vi "Create All Message Queues.vi"(8 "error in (no error)":errorcluster, 10 "Master Queue In":refnum<queue>) -> (0 "error out":errorcluster, 3 "Message Queues out":T1)   [LabVIEW 2013, in "MeasurementControl Message Queue.lvlib"]
doc: "This VI creates and initializes all the message queues for your application. If your application requires more than one message queue, right-click the \"Message Queues\" constant above and select Open Type Def. Add the new Message Queue(s) to the type definition, then initialize them in this VI."
uses:
  MeasurementControl Message Queue.lvlib
  All Message Queues.ctl
  Message Cluster.ctl
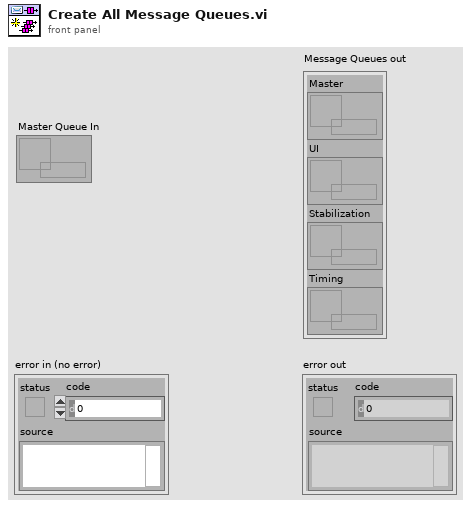
[diagram p1: front panel]
types:
  T1 = typedef "MeasurementControl Message Queue.lvlib/All Message Queues.ctl" = cluster{"Master":refnum<queue>, "UI":refnum<queue>, "Stabilization":refnum<queue>, "Timing":refnum<queue>}
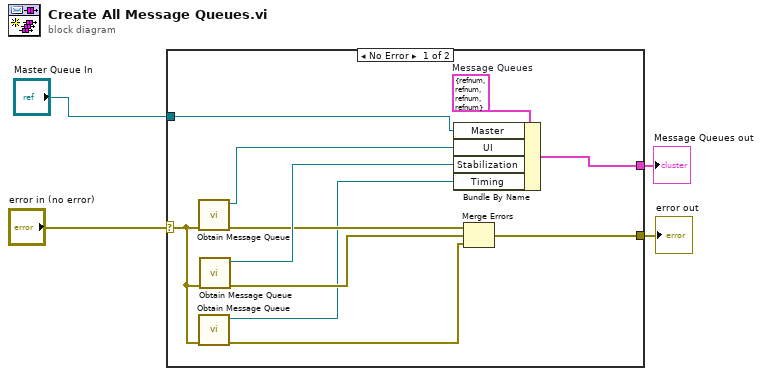
[diagram p0: block diagram]
diagram:
  n1 = case shown="No Error" "error in (no error)" {
    selector: "error in (no error)" -> [w7 w16]
    tunnel: [w13 w16] -> w4
    tunnel: [w14 _] -> w3
    tunnel: "Master Queue In" -> [w12 _]
    frame No Error {
      w15 = T1 {"Master"=refnum, "UI"=refnum, "Stabilization"=refnum, "Timing"=refnum}  # Message Queues
      n2 = call "Obtain Message Queue.vi"("error in (no error)"=w7) -> ("error out"=w9:errorcluster, "Message Queue"=w10:refnum<queue>)  [unwired: 9 in]
      n3 = call "Obtain Message Queue.vi"("error in (no error)"=w7) -> ("error out"=w5:errorcluster, "Message Queue"=w6:refnum<queue>)  [unwired: 9 in]
      n4 = call "Obtain Message Queue.vi"("error in (no error)"=w7) -> ("error out"=w8:errorcluster, "Message Queue"=w11:refnum<queue>)  [unwired: 9 in]
      n5 = Bundle By Name(cluster=w15, "Master"=w12, "UI"=w10, "Stabilization"=w11, "Timing"=w6) -> (w14:T1)
      n6 = Merge Errors(w9, w8, w5) -> (w13:errorcluster)
    }
    frame Error {
    }
  }
  "Message Queues out" <- w3
  "error out" <- w4
